vi "Host main.vi"() -> ()   [LabVIEW 2013]
uses:
  <vilib>/userdefined/High Color/nirio_resource_hc.ctl
  FPGA/DataMode.ctl
  <vilib>/FPGAPlugInAG/PXIe-7975R/niLvFpga_Open_PXIe-7975R.vi
  <vilib>/rvi/interface/common/dynamic/niFpgaDynamicAddResources.vi
  <vilib>/rvi/interface/common/niFpgaWaitOnOcc.vi
  <vilib>/Utility/error.llb/Error Cluster From Error Code.vi
  <vilib>/rvi/errors/niLvFpgaAdjustHostInterfaceError.vi
  <vilib>/FPGAPlugInAG/Dynamic/niLvFpga_Close_Dynamic.vi
  <vilib>/rvi/interface/nirviOpenFPGA/nirviOpenFPGA.xnode
  FPGA Bitfiles/mixer_FPGATarget_FPGAmain_cNAmzVB6sas.lvbitx
  <vilib>/rvi/interface/nirviReadWriteControl/nirviReadWriteControl.xnode
  <vilib>/rvi/interface/nirviMethod/nirviMethod.xnode
  <vilib>/rvi/interface/nirviCloseFPGA/nirviCloseFPGA.xnode
  NiFpgaLv.dll
  <vilib>/rvi/interface/Simulation/niFpgaSimulationCallBeginRW.vi
  <vilib>/FPGAPlugInAG/Dynamic/niLvFpga_ReadFifo_Dynamic.vi
  <vilib>/rvi/errors/niLvFpgaMergeErrorWithErrorCode.vi
panel:
  out "error IO":errorcluster
  out "CH1 Q":i16[](graph)
  out "CH1 I":i16[](graph)
  out "CH0 Q":i16[](graph)
  out "CH0 I":i16[](graph)
  in  "Sample":bool
  in  "Samples to aqcuire":u32
  in  "Mode":T1
  in  "stop":bool
  in  "Mixer requency [MHz]":dbl
  in  "resource name":T2
  out "Clocking Option Configured?":bool
  out "Configured?":bool
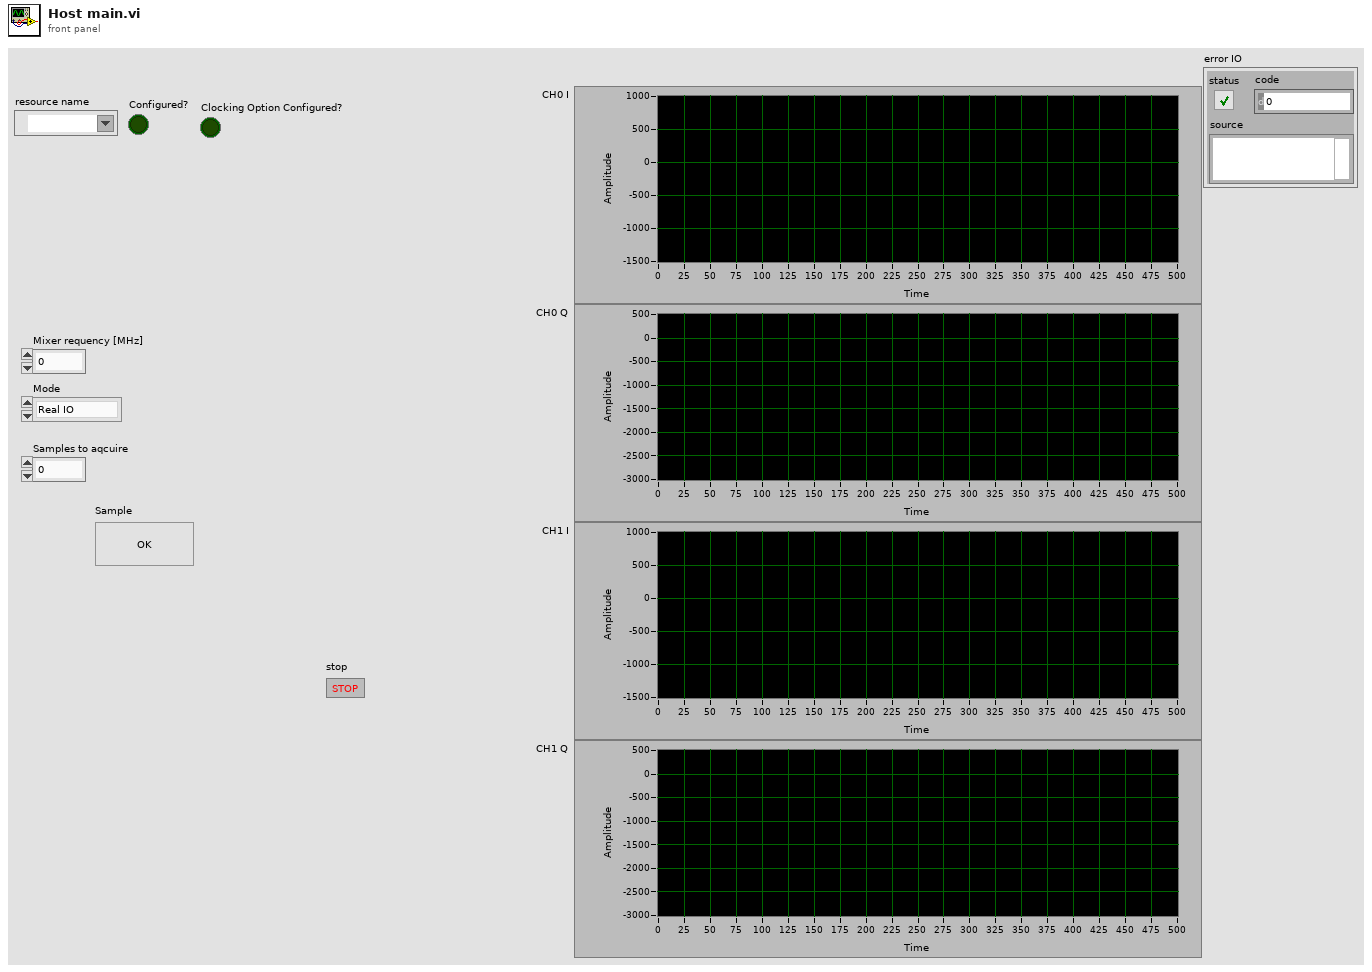
[diagram p1: front panel]
types:
  T1 = typedef "DataMode.ctl" = enum16{"Real IO", "Simulated"}
  T2 = typedef "nirio_resource_hc.ctl" = tag
  T3 = enum8{"Internal Clock PLL Off", "Internal Clock PLL On (REF IN)", "External Clock (CLK_IN)", "Internal Clock PLL On (IoModSyncClk)"}
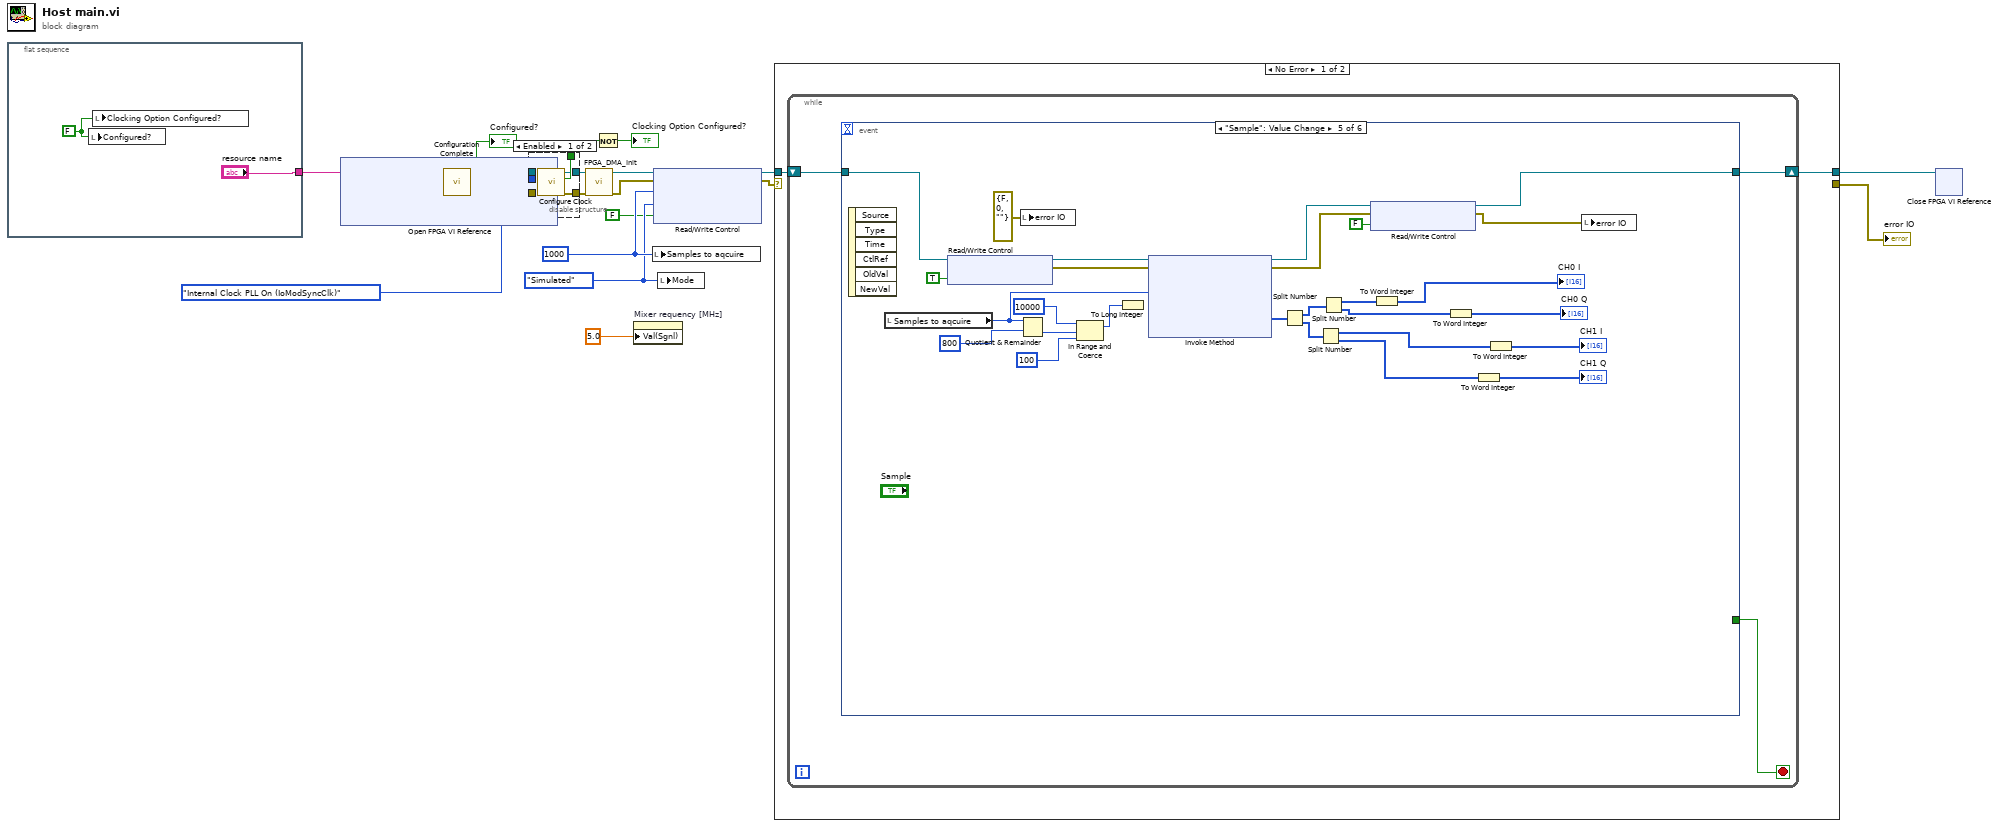
[diagram p0: block diagram]
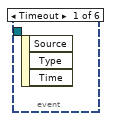
[diagram p3: hidden frame]
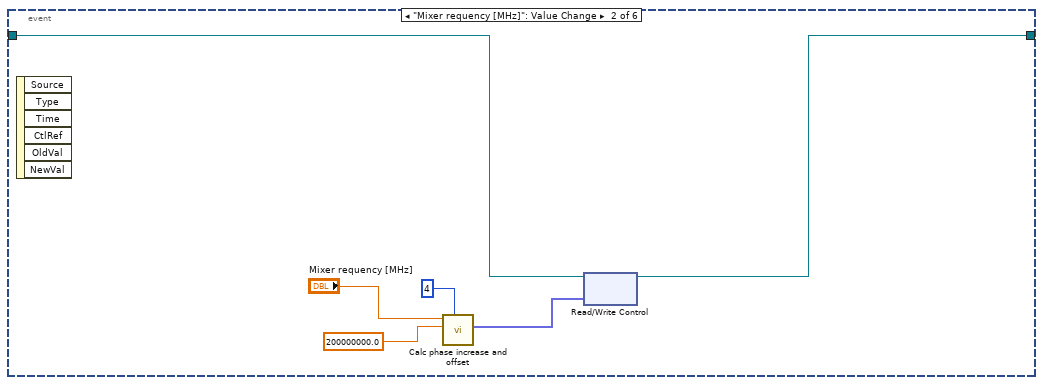
[diagram p4: hidden frame]
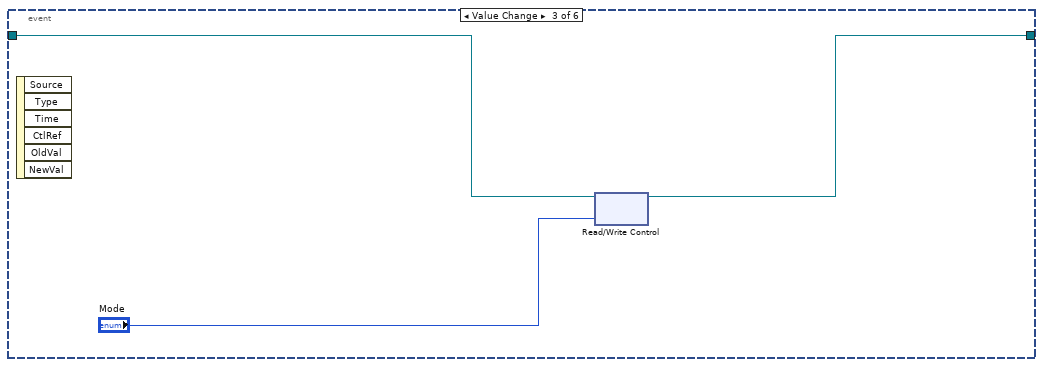
[diagram p5: hidden frame]
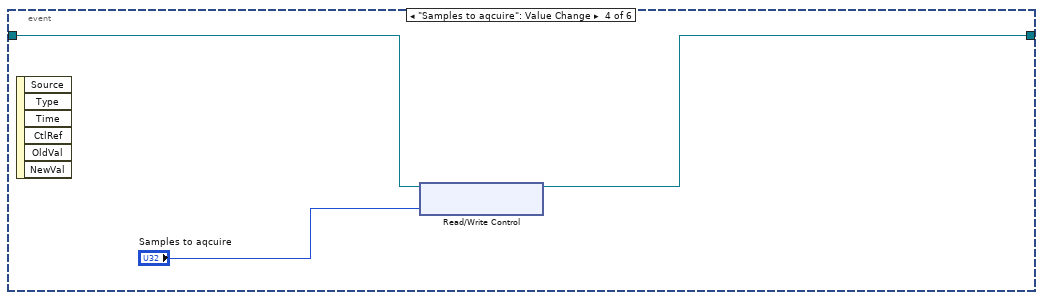
[diagram p6: hidden frame]
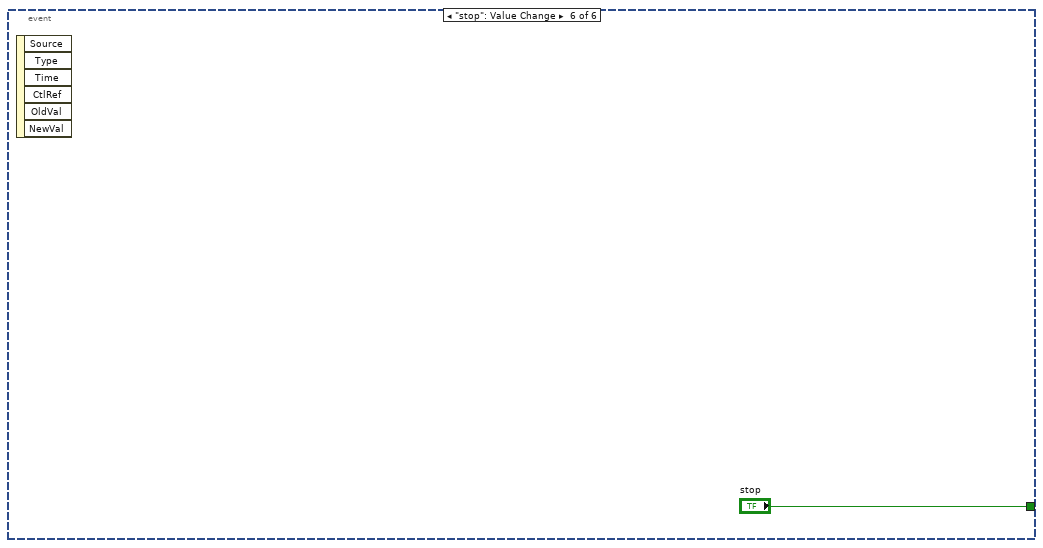
[diagram p7: hidden frame]
diagram:
  w9 = DataMode."Simulated" ("Mode")
  w10 = u32 1000 ("Samples to aqcuire")
  n1 = flat-sequence {
    tunnel: ["resource name"] -> w20
    frame #0 {
      w22 = FALSE ("Trigger Acquisition")
      n2 = local write "Configured?"(w22) -> ()
      n3 = local write "Clocking Option Configured?"(w22) -> ()
    }
  }
  n4 = xnode "Open FPGA VI Reference"("resource name"=w20) -> ("FPGA VI Reference Out"=w19:refnum<k20>, "error out"=w6:errorcluster)  [unwired: 1 in]
  n5 = call "Configuration Complete.vi"("error in"=w6, "FPGA VI Reference in"=w19) -> ("error out"=w5:errorcluster, "Configured?"=→"Configured?":bool, "FPGA VI Reference Out"=w18:refnum<k20>)  [unwired: 7 in]
  n6 = disable-structure shown="Enabled" {
    disable-tunnel: w18 -> [w29 w31]
    disable-tunnel: [w28 _] -> w16
    disable-tunnel: T3."Internal Clock PLL On (IoModSyncClk)" ("Clock Source") -> [w27 _]
    disable-tunnel: [w26 w31] -> w13
    disable-tunnel: w5 -> [w25 w30]
    disable-tunnel: [w24 w30] -> w4
    frame Enabled {
      n7 = call "Configure Clock.vi"("error in"=w25, "Clock Source"=w27, "FPGA VI Reference in"=w29) -> ("error out"=w24:errorcluster, "Configuration Error"=w28:bool, "FPGA VI Reference Out"=w26:refnum<k20>)  [unwired: 6 in]
    }
    frame Disabled {
    }
  }
  n8 = call "FPGA_DMA_Init.vi"("error in (no error)"=w4, "FPGA VI Reference"=w13) -> ("error out"=w3:errorcluster, "FPGA VI out"=w12:refnum<k20>)  [unwired: 7 in, 1 out]
  n9 = Not(x=w16) -> (.not. x?=→"Clocking Option Configured?":bool)
  n10 = property on="Mixer requency [MHz]" class="DigNum (strict)"("Val(Sgnl)"=5.0 ("Mixer requency [MHz]")) -> ()  [unwired: 2 in, 2 out]
  n11 = local write "Samples to aqcuire"(w10) -> ()
  n12 = xnode "Read/Write Control"("FPGA VI Reference In"=w12, "error in"=w3, "Samples Per Trigger"=w10, "Mode"=w9, "Trigger Acquisition"=FALSE) -> ("FPGA VI Reference Out"=w11:refnum<k20>, "error out"=w2:errorcluster)
  n13 = local write "Mode"(w9) -> ()
  n14 = case shown="No Error" w2 {
    selector: w2 -> [_ w77]
    tunnel: [w33 w78] -> w14
    tunnel: w11 -> [w32 w78]
    tunnel: [_ w77] -> w1
    frame No Error {
      n15 = while {
        shift-right: [w35] -> w33
        shift-left: w32 -> [w36]
        stop <- w34 stop-if-true
        n16 = event shown="[4] \"Sample\": Value Change" {
          selector: _ -> [_ _ _ _ _ _]
          dyn-events: _ -> [_ _ _ _ _ _]
          timeout: _ -> [_ _ _ _ _ _]
          tunnel: w36 -> [_ w40 w45 w48 w75 _]
          tunnel: [_ w39 w44 w47 w63 _] -> w35
          tunnel: [_ _ _ _ _ "stop"] -> w34
          event Timeout {
            n17 = event-data() -> ()  [unwired: 1 in, 3 out]
          }
          event "Mixer requency [MHz]": Value Change {
            n18 = event-data() -> ()  [unwired: 1 in, 6 out]
            n19 = call "Calc phase increase and offset.vi"("# of DDS"=4, "fclk (800MHz)"=200000000.0, "f_generated (MHz)"="Mixer requency [MHz]") -> ("Phase out"=w38:fxp<+,64,64>[])  [unwired: 6 in, 2 out]
            n20 = xnode "Read/Write Control"("FPGA VI Reference In"=w40, "Phase"=w38) -> ("FPGA VI Reference Out"=w39:refnum<k20>)  [unwired: 1 in, 1 out]
          }
          event Value Change {
            n21 = event-data() -> ()  [unwired: 1 in, 6 out]
            n22 = xnode "Read/Write Control"("FPGA VI Reference In"=w45, "Mode"="Mode") -> ("FPGA VI Reference Out"=w44:refnum<k20>)  [unwired: 1 in, 1 out]
          }
          event "Samples to aqcuire": Value Change {
            n23 = event-data() -> ()  [unwired: 1 in, 6 out]
            n24 = xnode "Read/Write Control"("FPGA VI Reference In"=w48, "Samples Per Trigger"="Samples to aqcuire") -> ("FPGA VI Reference Out"=w47:refnum<k20>)  [unwired: 1 in, 1 out]
          }
          event "Sample": Value Change {
            n25 = event-data() -> ()  [unwired: 1 in, 6 out]
            n26 = local read "Samples to aqcuire"() -> (w62:u32)
            n27 = xnode "Read/Write Control"("FPGA VI Reference In"=w75, "Trigger Acquisition"=TRUE) -> ("FPGA VI Reference Out"=w73:refnum<k20>, "error out"=w56:errorcluster)  [unwired: 1 in]
            n28 = Quotient & Remainder(x=w62, y=u32 800) -> (floor(x/y)=w60:u32)  [unwired: 1 out]
            n29 = local write "error IO"(errorcluster {"status"=FALSE, "code"=0, "source"=""} ("error IO")) -> ()
            n30 = In Range and Coerce(upper limit=u32 10000, x=w60, lower limit=u32 100) -> (coerced(x)=w57:u32)  [unwired: 1 out]
            n31 = To Long Integer(number=w57) -> ()  [unwired: 1 out]
            n32 = xnode "Invoke Method"("FPGA VI Reference In"=w73, "error in"=w56, "Number of Elements"=w62) -> ("FPGA VI Reference Out"=w64:refnum<k20>, "error out"=w55:errorcluster, "Data"=w70:u64[])  [unwired: 1 in, 1 out]
            n33 = Split Number(x=w70) -> (hi(x)=w72:u32[], lo(x)=w71:u32[])
            n34 = Split Number(x=w71) -> (hi(x)=w68:u16[], lo(x)=w67:u16[])
            n35 = Split Number(x=w72) -> (hi(x)=w66:u16[], lo(x)=w69:u16[])
            n36 = xnode "Read/Write Control"("FPGA VI Reference In"=w64, "error in"=w55, "Trigger Acquisition"=FALSE) -> ("FPGA VI Reference Out"=w63:refnum<k20>, "error out"=w54:errorcluster)
            n37 = To Word Integer(number=w66) -> (16bit integer=→"CH0 I":i16[])
            n38 = To Word Integer(number=w69) -> (16bit integer=→"CH0 Q":i16[])
            n39 = To Word Integer(number=w67) -> (16bit integer=→"CH1 Q":i16[])
            n40 = To Word Integer(number=w68) -> (16bit integer=→"CH1 I":i16[])
            n41 = local write "error IO"(w54) -> ()
          }
          event "stop": Value Change {
            n42 = event-data() -> ()  [unwired: 1 in, 6 out]
          }
        }
      }
    }
    frame Error {
    }
  }
  "error IO" <- w1
  n43 = xnode "Close FPGA VI Reference"("FPGA VI Reference In"=w14) -> ()  [unwired: 1 in, 1 out]
